vi "Matrix_read_target.vi"   [LabVIEW 2018]
uses:
  <vilib>/platform/TimedLoop/XDataNode/XDataNode.xnode
  <vilib>/Platform/TimedLoop/XDataNode/nitl_modes.ctl
  <vilib>/Platform/TimedLoop/XDataNode/XDNodeRunTimeDep.lvlib
  <vilib>/Platform/TimedLoop/XDataNode/wakeup.ctl
  <vilib>/Platform/TimedLoop/XDataNode/timing_clust.ctl
  <vilib>/eio/EIONode/EIONode.xnode
  <vilib>/rvi/eio/common/nirviEmuTemplateMethod_errors.vi
types:
  T1 = typedef "XDNodeRunTimeDep.lvlib/timing_clust.ctl" = cluster{"Expected End [f-1]":u64, "Actual End [f-1]":u64, "Finished Late? [f-1]":bool, "Expected End [i-1]":u64, "Actual End [i-1]":u64, "Finished Late? [i-1]":bool, "Expected Start [i]":u64, "Actual Start [i]":u64, "Expected Start [f]":u64, "Actual Start [f]":u64, "Source Name":string, "Structure Name":string, "Period":i64, "Deadline":i64, "Offset":i64, "Start":i64, "Priority":i32, "Timeout":i32, "Mode":T2, "Wakeup Reason":T3, "Error":errorcluster, "Source Type":string, "Secondary Source Type":string, "Global End Time":u64, "Global Start Time":u64, "Frame Duration":u64, "Iteration Duration":u64, "Assigned CPU":i32, "I/O Scan Engine Mode":u32}
  T2 = typedef "XDNodeRunTimeDep.lvlib/nitl_modes.ctl" = enum32{"No Change", "Process missed periods, maintain original phase", "Discard missed periods, maintain original phase", "Process missed periods, ignore original phase", "Discard missed periods, ignore original phase"}
  T3 = typedef "XDNodeRunTimeDep.lvlib/wakeup.ctl" = enum32{"Normal", "Aborted", "Asynchronous wakeup", "Timing source error", "Timed loop error", "Timeout"}
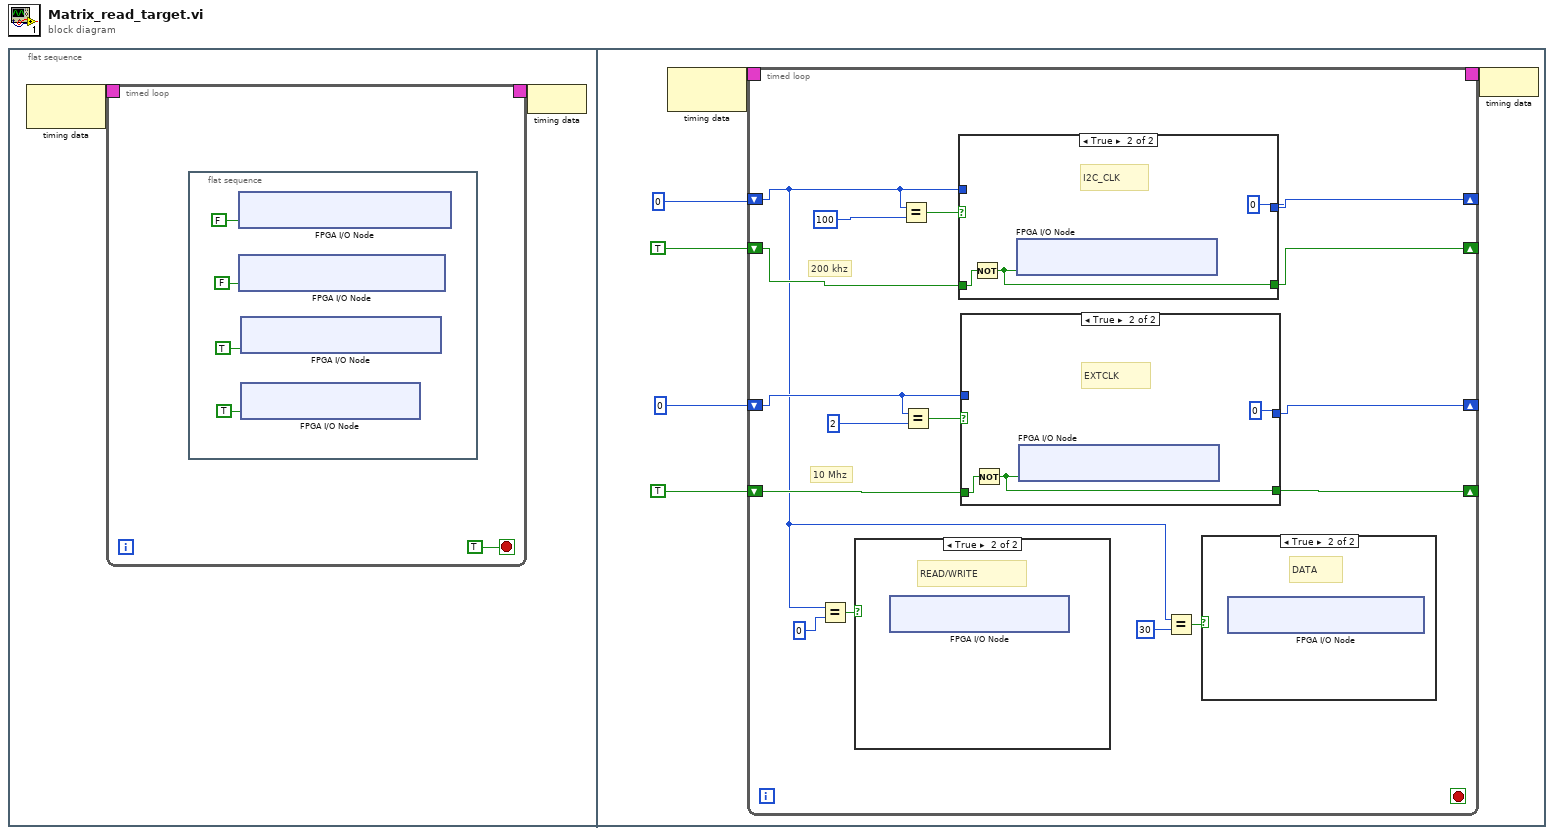
[diagram p0: block diagram]
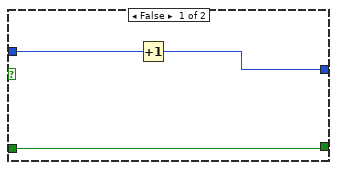
[diagram p4: hidden frame]
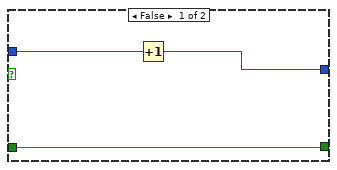
[diagram p5: hidden frame]
diagram:
  n1 = flat-sequence {
    frame #0 {
      n2 = node-c288() -> (w2:T1)  [unwired: 1 in]
      n3 = timed-loop {
        timing: w2 -> [_]
        timing-out: [_] -> w1
        stop <- TRUE stop-if-true
        n4 = flat-sequence {
          frame #0 {
            n5 = xnode "FPGA I/O Node"("IO Module\\DDCA_DIO16-23_WE"=FALSE ("IO Module\\DDCA_DIO16-23_WE")) -> ()  [unwired: 1 in, 1 out]
            n6 = xnode "FPGA I/O Node"("IO Module\\DDCA_DIO8-15_WE"=FALSE ("IO Module\\DDCA_DIO8-15_WE")) -> ()  [unwired: 1 in, 1 out]
            n7 = xnode "FPGA I/O Node"("IO Module\\DDCA_DIO0-7_WE"=TRUE ("IO Module\\DDCA_DIO0-7_WE")) -> ()  [unwired: 1 in, 1 out]
            n8 = xnode "FPGA I/O Node"("IO Module\\DDCA_PFI_WE"=TRUE ("IO Module\\DDCA_DIO0-7_WE")) -> ()  [unwired: 1 in, 1 out]
          }
        }
      }
      n9 = node-c288(w1) -> ()
    }
    frame #1 {
      n10 = node-c288() -> (w17:T1)  [unwired: 1 in]
      n11 = timed-loop {
        timing: w17 -> [_]
        timing-out: [_] -> w16
        shift-right: [w31] -> _
        shift-left: 0 -> [w20]
        shift-right: [w30] -> _
        shift-left: 0 -> [w27]
        shift-right: [w23] -> _
        shift-left: TRUE -> [w24]
        shift-right: [w25] -> _
        shift-left: TRUE -> [w26]
        stop <- _ stop-if-true
        # "10 Mhz"
        # "200 khz"
        n12 = Equal?(x=w20, y=0) -> (x = y?=w22:bool)
        n13 = case shown="True" w22 {
          frame False {
          }
          frame True {
            # "READ/WRITE"
            n14 = xnode "FPGA I/O Node"() -> ()  [unwired: 2 in, 1 out]
          }
        }
        n15 = Equal?(x=w20, y=100 ("100")) -> (x = y?=w33:bool)
        n16 = Equal?(x=w27, y=2 ("100")) -> (x = y?=w28:bool)
        n17 = case shown="True" w33 {
          tunnel: [w41 0] -> w31
          tunnel: w20 -> [w42 _]
          tunnel: [w40 w44] -> w25
          tunnel: w26 -> [w40 w43]
          frame False {
            n18 = Increment(x=w42) -> (x+1=w41:i32)
          }
          frame True {
            # "I2C_CLK"
            n19 = Not(x=w43) -> (.not. x?=w44:bool)
            n20 = xnode "FPGA I/O Node"("IO Module\\DDCA_DIO6_Write"=w44) -> ()  [unwired: 1 in, 1 out]
          }
        }
        n21 = case shown="True" w28 {
          tunnel: [w35 0] -> w30
          tunnel: w27 -> [w36 _]
          tunnel: [w34 w38] -> w23
          tunnel: w24 -> [w34 w37]
          frame False {
            n22 = Increment(x=w36) -> (x+1=w35:i32)
          }
          frame True {
            # "EXTCLK"
            n23 = Not(x=w37) -> (.not. x?=w38:bool)
            n24 = xnode "FPGA I/O Node"("IO Module\\DDCA_DIO7_Write"=w38) -> ()  [unwired: 1 in, 1 out]
          }
        }
        n25 = Equal?(x=w20, y=30) -> (x = y?=w21:bool)
        n26 = case shown="True" w21 {
          frame False {
          }
          frame True {
            # "DATA"
            n27 = xnode "FPGA I/O Node"() -> ()  [unwired: 2 in, 1 out]
          }
        }
      }
      n28 = node-c288(w16) -> ()
    }
  }
